vi "Periodic Tasks.vi"(8 "error in":errorcluster) -> ()   [LabVIEW 2020]
doc: "This VI runs in parallel to other tasks. It can contain as many user-defined periodic loops as you need. These can carry out PID or other sorts of timed response."
uses:
  <vilib>/Rock Robotics/WPI/Relay/WPI_RelayValue.ctl
  <vilib>/Rock Robotics/WPI/Utilities/WPI_GetSetVariantRefNum.vi
  <vilib>/Rock Robotics/Network Tables/NT Write Boolean.vi
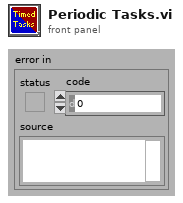
[diagram p1: front panel]
types:
  T1 = typedef "WPI_RelayDevRef.ctl" = cluster{"DevStatus":errorcluster, "Relay Channel":T2, "Relay Direction":T3}
  T2 = typedef "FPGA_DIORelayChannel.ctl" = enum8{"Relay 0", "Relay 1", "Relay 2", "Relay 3", "Invalid"}
  T3 = typedef "WPI_RelayDirection.ctl" = enum16{"Both directions", "Forward only", "Reverse only"}
  T4 = typedef "WPI_SwitchDevRef.ctl" = cluster{"DevStatus":errorcluster, "DIO Channel":T5, "CntIndex":T6, "Normally Closed":bool}
  T5 = typedef "FPGA_DIOChannel.ctl" = enum8{"DIO 0", "DIO 1", "DIO 2", "DIO 3", "DIO 4", "DIO 5", "DIO 6", "DIO 7", "DIO 8", "DIO 9", "DIO MXP 0", "DIO MXP 1", "DIO MXP 2", "DIO MXP 3", "DIO MXP 4", "DIO MXP 5", "DIO MXP 6", "DIO MXP 7", "DIO MXP 8", "DIO MXP 9", "DIO MXP 10", "DIO MXP 11", "DIO MXP 12", "DIO MXP 13", "DIO MXP 14", "DIO MXP 15", "SPI Port CS1", "SPI Port CS2", "SPI Port CS3", "SPI Port MISO", "SPI Port MOSI", "Invalid"}
  T6 = typedef "FPGA_CounterCtrSystemIndex.ctl" = enum8{"Ctr 0", "Ctr 1", "Ctr 2", "Ctr 3", "Ctr 4", "Ctr 5", "Ctr 6", "Ctr 7", "Invalid"}
  T7 = typedef "WPI_RelayValue.ctl" = enum16{"Off", "On", "Forward", "Reverse"}
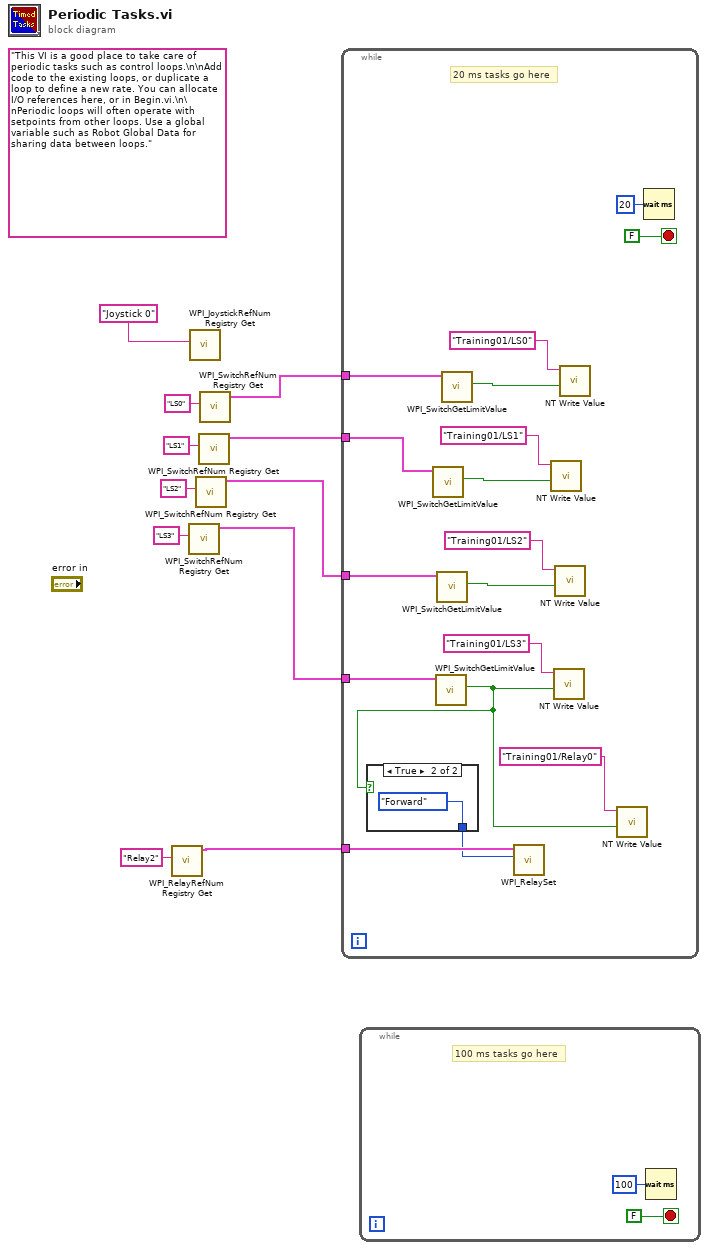
[diagram p0: block diagram]
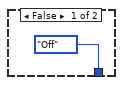
[diagram p2: hidden frame]
diagram:
  (unwired) "This VI is a good place to take care of periodic tasks such as control loops.\n\nAdd code to the existing loops, or duplicate a loop to define a new rate. You can allocate I/O references here, or in Begin.vi.\n\nPeriodic loops will often operate with setpoints from other loops. Use a global variable such as Robot Global Data for sharing data between loops."
  n1 = call <vilib>:"WPI_RelayRefNum Registry Get.vi"("refnum name"="Relay2") -> ("RelayDevRef"=w2:T1)  [unwired: 9 in, 1 out]
  n2 = call <vilib>:"WPI_SwitchRefNum Registry Get.vi"("refnum name"="LS3") -> ("SwitchDevRef"=w3:T4)  [unwired: 9 in, 1 out]
  n3 = call <vilib>:"WPI_JoystickRefNum Registry Get.vi"("refnum name"="Joystick 0") -> ()  [unwired: 1 in, 10 out]
  n4 = call <vilib>:"WPI_SwitchRefNum Registry Get.vi"("refnum name"="LS2") -> ("SwitchDevRef"=w4:T4)  [unwired: 9 in, 1 out]
  n5 = call <vilib>:"WPI_SwitchRefNum Registry Get.vi"("refnum name"="LS1") -> ("SwitchDevRef"=w5:T4)  [unwired: 9 in, 1 out]
  n6 = call <vilib>:"WPI_SwitchRefNum Registry Get.vi"("refnum name"="LS0") -> ("SwitchDevRef"=w6:T4)  [unwired: 9 in, 1 out]
  n7 = while {
    tunnel: w6 -> [w26]
    tunnel: w5 -> [w18]
    tunnel: w4 -> [w17]
    tunnel: w3 -> [w16]
    tunnel: w2 -> [w14]
    stop <- FALSE stop-if-true
    # "20 ms tasks go here"
    n8 = call <vilib>:"WPI_SwitchGetLimitValue.vi"("SwitchDevRef"=w18) -> ("Switch Pressed"=w22:bool)  [unwired: 8 in, 2 out]
    n9 = call <vilib>:"WPI_SwitchGetLimitValue.vi"("SwitchDevRef"=w16) -> ("Switch Pressed"=w13:bool)  [unwired: 8 in, 2 out]
    n10 = case shown="True" w13 {
      tunnel: [WPI_RelayValue."Off" ("RelayValue") WPI_RelayValue."Forward" ("RelayValue")] -> w12
      frame False {
      }
      frame True {
      }
    }
    n11 = call <vilib>:"WPI_SwitchGetLimitValue.vi"("SwitchDevRef"=w17) -> ("Switch Pressed"=w20:bool)  [unwired: 8 in, 2 out]
    n12 = call <vilib>:"WPI_SwitchGetLimitValue.vi"("SwitchDevRef"=w26) -> ("Switch Pressed"=w24:bool)  [unwired: 8 in, 2 out]
    n13 = call <vilib>:"WPI_RelaySet.vi"("RelayValue"=w12, "RelayDevRef"=w14) -> ()  [unwired: 8 in, 2 out]
    n14 = call-poly <vilib>:"NT Write Value.vi"("value"=w22, "name"="Training01/LS1") -> ()  [unwired: 9 in, 1 out]
    n15 = call-poly <vilib>:"NT Write Value.vi"("value"=w13, "name"="Training01/LS3") -> ()  [unwired: 9 in, 1 out]
    n16 = call-poly <vilib>:"NT Write Value.vi"("value"=w20, "name"="Training01/LS2") -> ()  [unwired: 9 in, 1 out]
    n17 = call-poly <vilib>:"NT Write Value.vi"("value"=w24, "name"="Training01/LS0") -> ()  [unwired: 9 in, 1 out]
    n18 = call-poly <vilib>:"NT Write Value.vi"("value"=w13, "name"="Training01/Relay0") -> ()  [unwired: 9 in, 1 out]
    n19 = Wait (ms)(milliseconds to wait=u32 20) -> ()  [unwired: 1 out]
  }
  n20 = while {
    stop <- FALSE stop-if-true
    # "100 ms tasks go here"
    n21 = Wait (ms)(milliseconds to wait=u32 100) -> ()  [unwired: 1 out]
  }
